vi "Connect.vi"(8 "error in":errorcluster, 10 "Additional Information":string, 11 "DB-ADO in":refnum<class "DB-ADO.lvclass">) -> (0 "error out":errorcluster, 3 "DB-ADO out":refnum<class "DB-ADO.lvclass">)   [LabVIEW 2014, in "hse-db.lvlib" / "DB-ADO.lvclass"]
doc: "Connect to a ADO database."
uses:
  DB-ADO.lvclass
  DB-Interface.lvclass/DB-Interface.ctl
  DB-ADO.lvclass/DB-ADO.ctl
  DB-Engines/ADO-DB-Drivers/ADO-DB-Driver.lvlib
  DB-Interface.lvclass
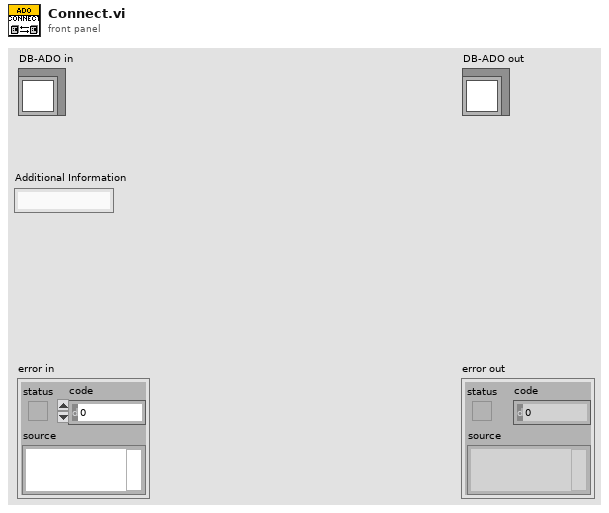
[diagram p1: front panel]
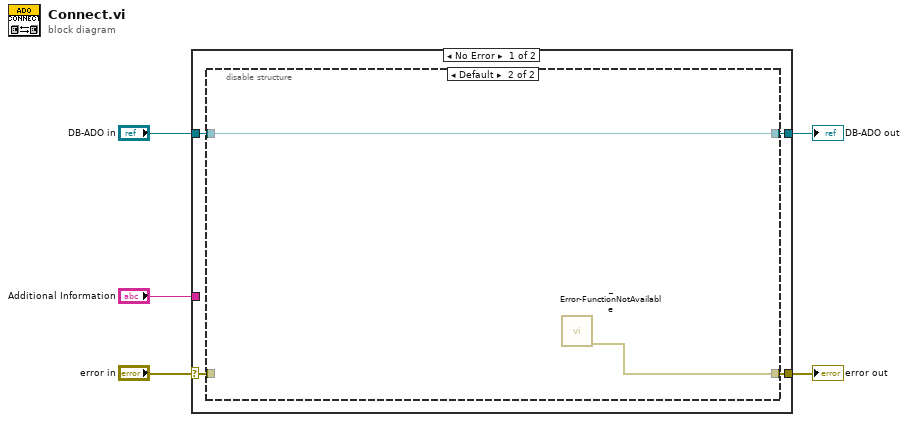
[diagram p0: block diagram]
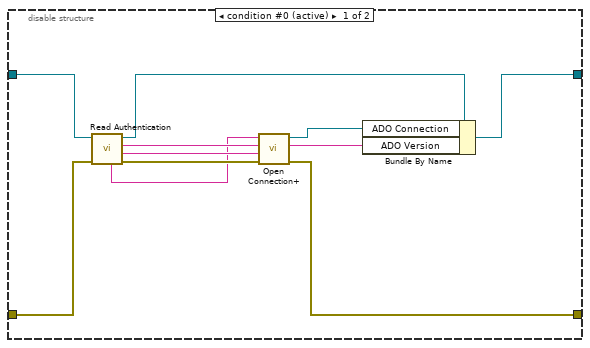
[diagram p2: hidden frame]
diagram:
  n1 = case shown="No Error" "error in" {
    selector: "error in" -> [w8 w24]
    tunnel: [w7 w24] -> w4
    tunnel: [w6 w23] -> w2
    tunnel: "DB-ADO in" -> [w9 w23]
    tunnel: "Additional Information" -> [_ _]
    frame No Error {
      n2 = disable-structure shown="Default" {
        disable-tunnel: w9 -> [w20 w22]
        disable-tunnel: w8 -> [w15 _]
        disable-tunnel: [w14 w21] -> w7
        disable-tunnel: [w11 w22] -> w6
        frame condition #0 (active) {
          n3 = call "Read Authentication.vi"("error in"=w15, "DB-Engine in"=w20) -> ("error out"=w17:errorcluster, "Password"=w18:string, "User"=w19:string, "DB-Engine out"=w12:refnum<class "DB-ADO.lvclass">, "Database"=w16:string)  [unwired: 5 in]
          n4 = call "Open Connection+.vi"("error in (no error)"=w17, "Password"=w18, "UserID"=w19, "Connection String"=w16) -> ("error out"=w14:errorcluster, "ADO Version"=w10:string, "Connection"=w13:refnum<k7>)  [unwired: 5 in]
          n5 = Bundle By Name(cluster=w12, "ADO Connection"=w13, "ADO Version"=w10) -> (w11:refnum<class "DB-ADO.lvclass">)
        }
        frame condition #1 {
          n6 = call "_Error-FunctionNotAvailable.vi"() -> ("error out"=w21:errorcluster)  [unwired: 11 in]
        }
      }
    }
    frame Error {
    }
  }
  "error out" <- w4
  "DB-ADO out" <- w2
